vi "Panel Dryer Wilt Details.vi"(0 "Dryer In":T4 {"Night Cycle Count" format="%04d"; "Dryer Details"."Stop Dryer" items=["NO", "YES"]; "Dryer Details"."24 Hour Water Injection" items=["NO", "YES"]; "Dryer Details"."Run w/o Newfi" items=["NO", "YES"]; "Day Cycle Count" format="%04d"}, 1 "FileName":path caption="Sample Datafilename", 9 "Test State":T2) -> (4 "Dryer Details Out":T3 {"Stop Dryer" items=["NO", "YES"]; "24 Hour Water Injection" items=["NO", "YES"]; "Run w/o Newfi" items=["NO", "YES"]}, 6 "New Filenames":bool, 8 "Updated":bool, 10 "Audit Alert Out":bool)   [LabVIEW 2012]
uses:
  Dryer.ctl
  Dryer Details.ctl
  Dryer Test State.ctl
  Globals Wilt.vi
panel:
  in  "Audit Alert Button":bool
  in  "Return":bool
  out "Time":dbl[](array[numeric])
  out "Cycle Count":dbl[](array[numeric])
  in  "Tab Control":T1(tab)
  out "Dryer Details":T3 {"Stop Dryer" items=["NO", "YES"]; "24 Hour Water Injection" items=["NO", "YES"]; "Run w/o Newfi" items=["NO", "YES"]}
  out "Total Cycle Count":i32
  out "Station Number":string
  out "Status Color":u32(colorbox)
  out "Bad Com Count":i32
  out "Com Port":u8
  out "Boolean":bool
  out "Audit Alert":bool
  out "Sample Plot":cluster{dbl[], dbl[]}[](graph)
  out "Current Cycle Count":dbl
  out "I(L1),I(L2),Trmb,V.V2":dbl[][](array[numeric])
  out "Cycle Count 2":dbl[](array[numeric])
  out "Completion time":dbl[](array[numeric])
  out "L1max":dbl[](array[numeric])
  out "L2max":dbl[](array[numeric])
  out "Tmax":dbl[](array[numeric])
  out "History Plot":cluster{dbl[], dbl[]}[](graph)
  out "Serial Com Array":cluster{dbl, string}[](array[cluster]) {"?" format="%<%H:%M:%S>t"}
  out "Voltage 2":dbl[](array[numeric])
  out "Voltage":dbl[](array[numeric])
  out "Trmb":dbl[](array[numeric])
  out "L2":dbl[](array[numeric])
  out "L1":dbl[](array[numeric])
  out "Sample Record":string[][](array[string])
  out "all rows":string[][](array[string])
  in  "Read Sample Record(t, CC, Tc, \nASCII, Status, L1,L2,Trmb,V{,V2,SW} )":string[][](array[string])
  in  "Update":bool
  # "D"
  # "N"
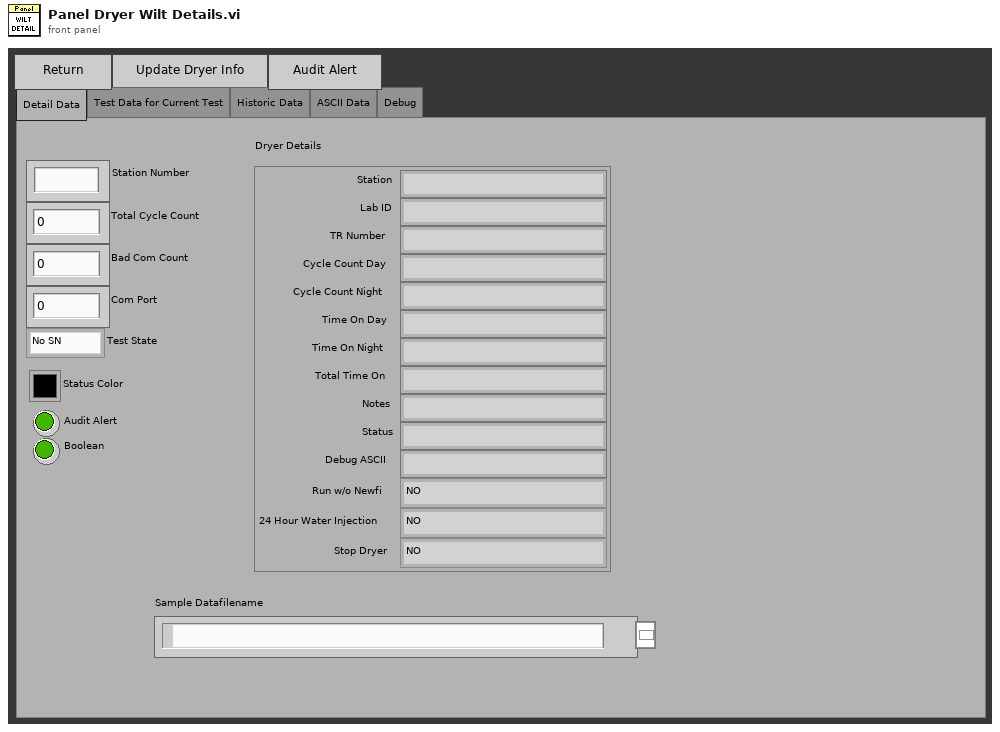
[diagram p1: front panel]
types:
  T1 = enum32{"Detail Data", "Test Data for Current Test", "Historic Data", "ASCII Data", "Debug"}
  T2 = typedef "Dryer Test State.ctl" = enum16{"No SN", "Wait Com", "Wait to Start", "Watering", "Drying", "Cooldown", "Paused", "Temp Fault", "Com Fault", "Pause Manual Station"}
  T3 = typedef "Dryer Details.ctl" = cluster{"Station":string, "Cycle Count Day":string, "Status":string, "Debug ASCII":string, "Notes":string, "Lab ID":string, "Total Time On":string, "TR Number":string, "Cycle Count Night":string, "Time On Day":string, "Time On Night":string, "Run w/o Newfi":i32, "24 Hour Water Injection":i32, "Stop Dryer":i32}
  T4 = typedef "Dryer.ctl" = cluster{"Lab ID":string, "Day Cycle Count":i32, "Station Label":string, "Dryer Details":T3, "Sample Record ":string[], "Hist Record ":string[][], "Status Color":u32, "Boolean":bool, "Com Port":u8, "Bad Com Count":i32, "Current Run Start Time":dbl, "Night Cycle Count":i32, "Station Index":i32, "Cycle Index":string, "Audit Alert":bool}
  T5 = enum16{"Read 2D Array", "Write 2D Array", "Write/Append 1D Array"}
  T6 = cluster{"FileName":path, "New File Info":bool, "Dryer In":T4, "Read Sample Record(t, CC, Tc, \nASCII, Status, L1,L2,Trmb,V{,V2,SW} )":string[][], "Audit Alert":bool, "Updated":bool}
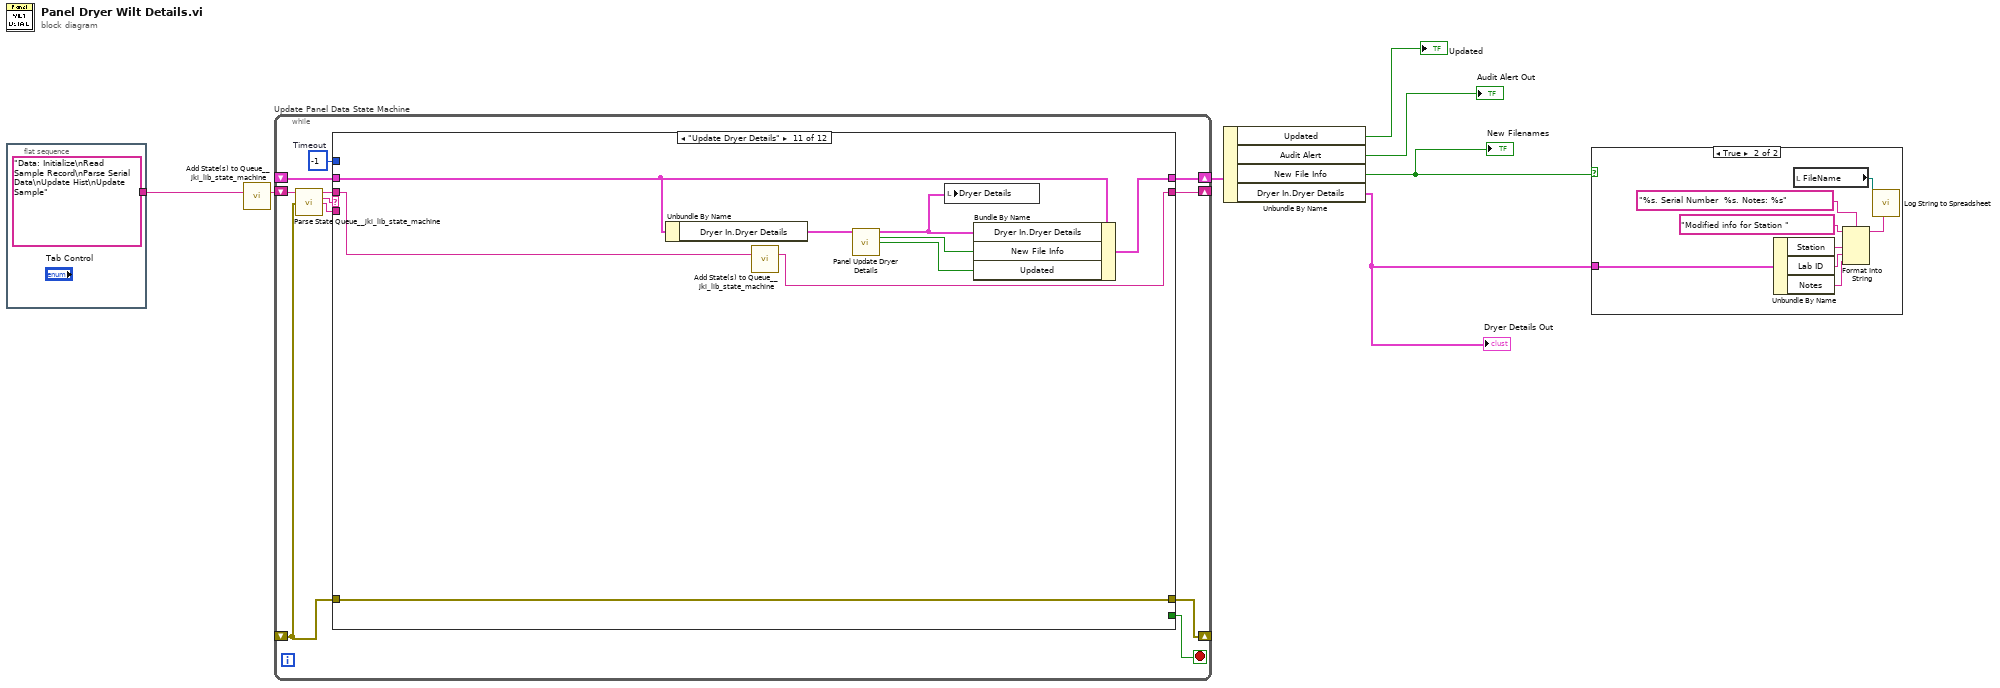
[diagram p0: block diagram]
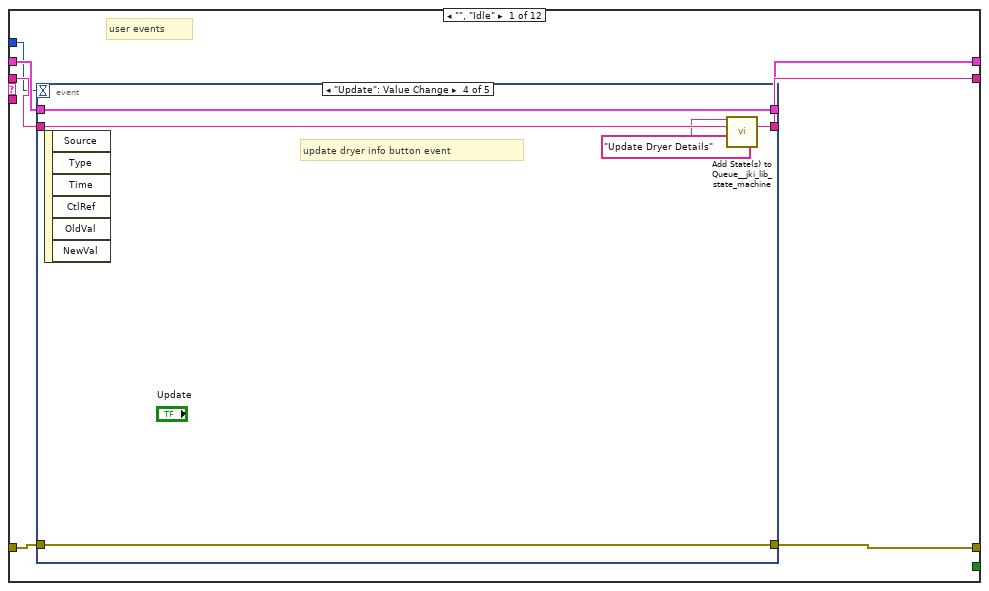
[diagram p2: hidden frame]
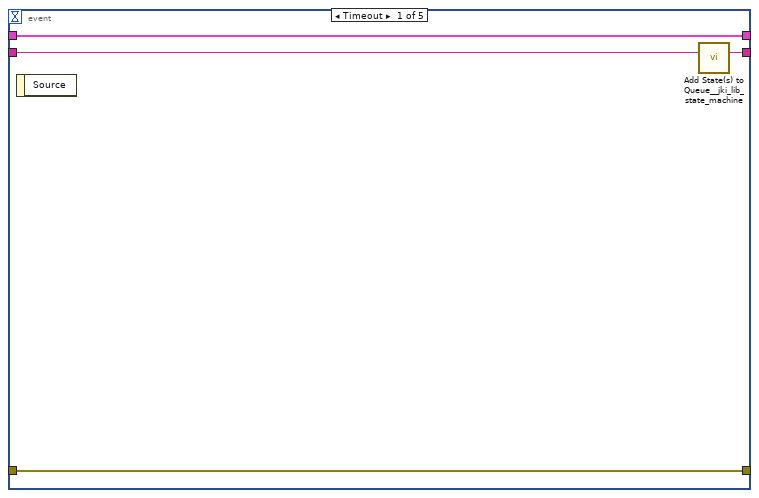
[diagram p3: hidden frame]
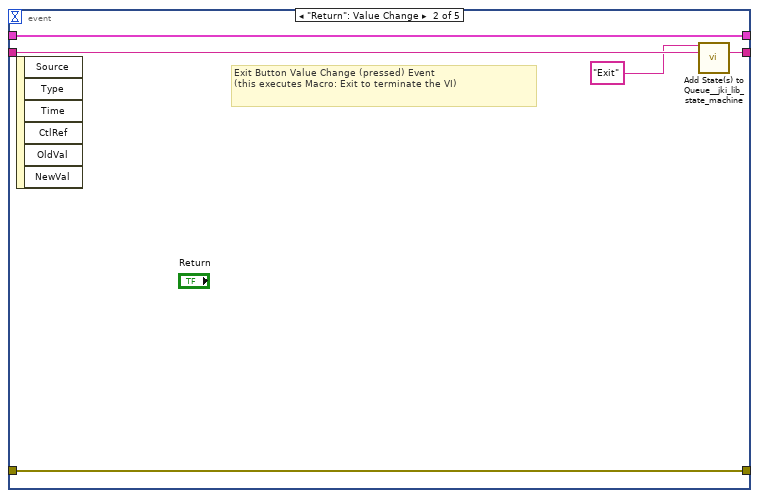
[diagram p4: hidden frame]
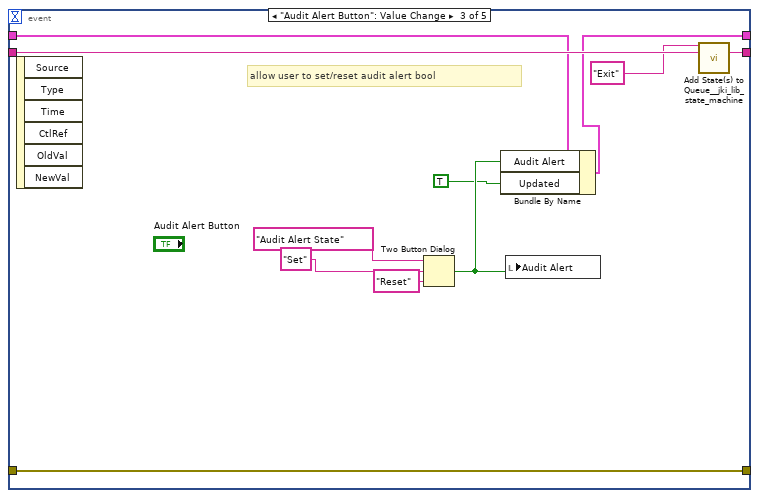
[diagram p5: hidden frame]
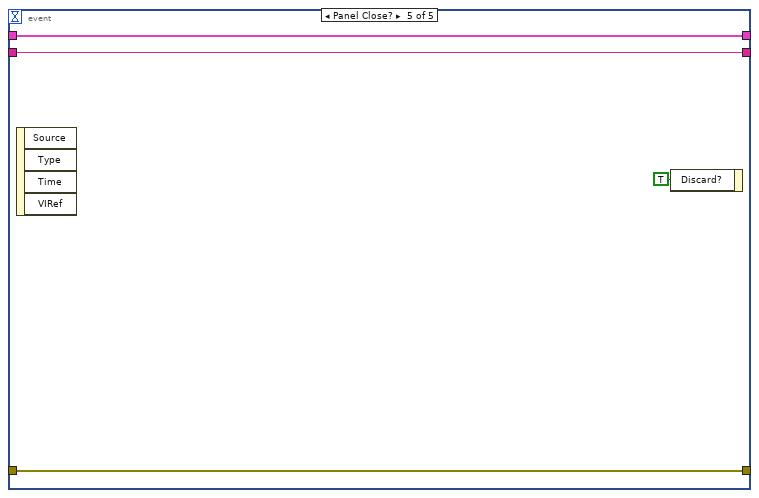
[diagram p6: hidden frame]
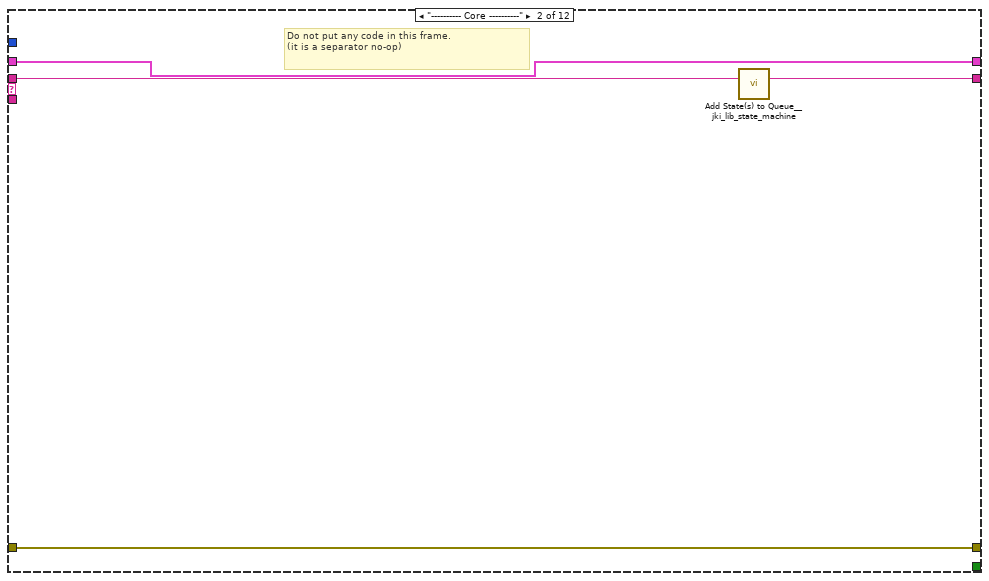
[diagram p7: hidden frame]
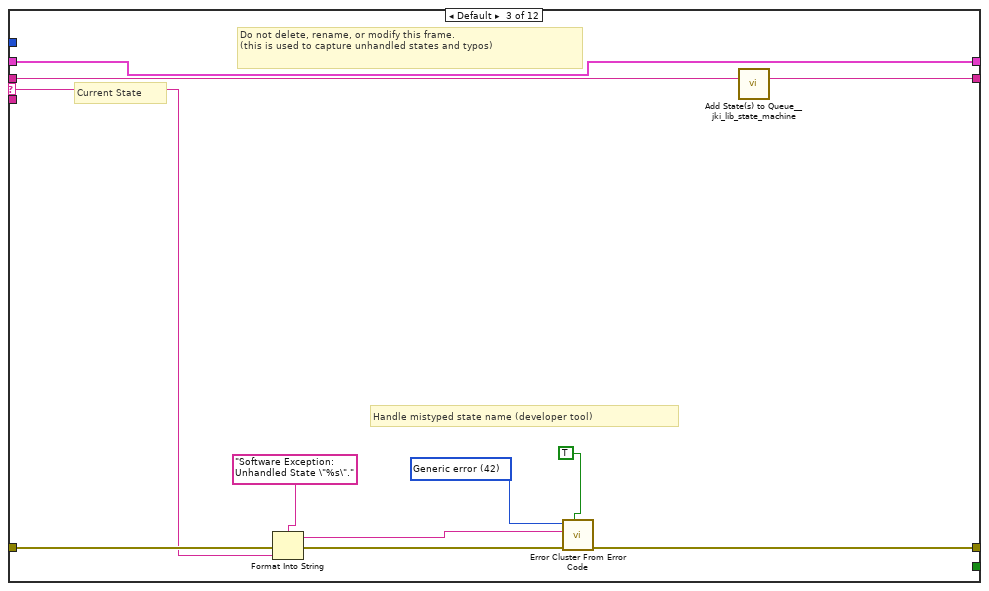
[diagram p8: hidden frame]
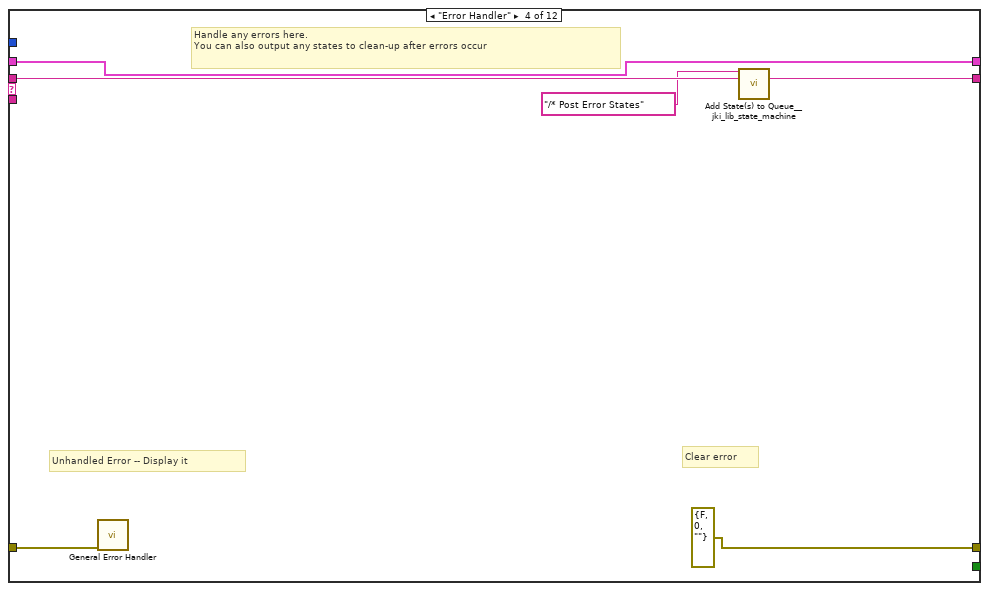
[diagram p9: hidden frame]
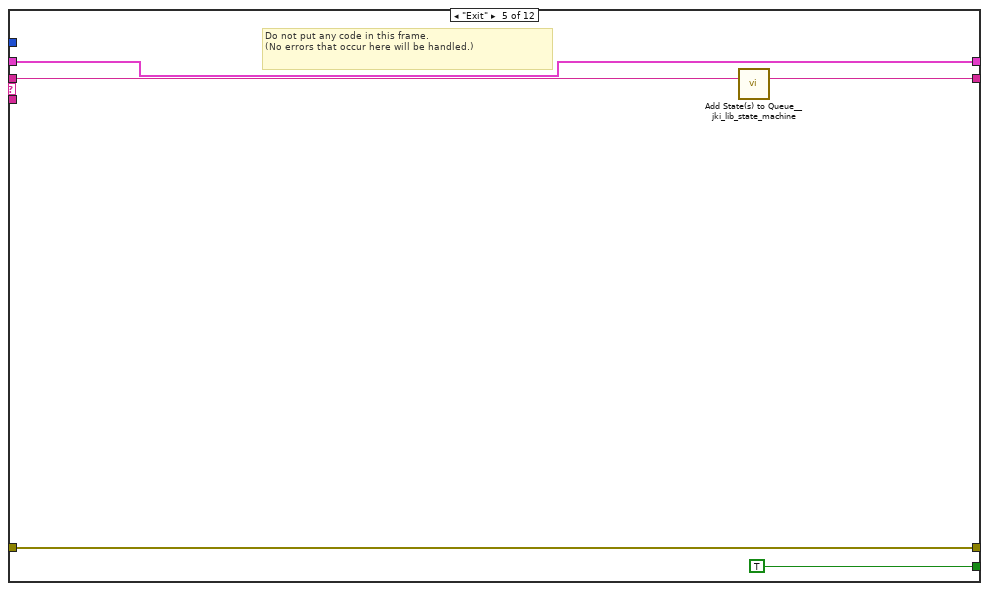
[diagram p10: hidden frame]
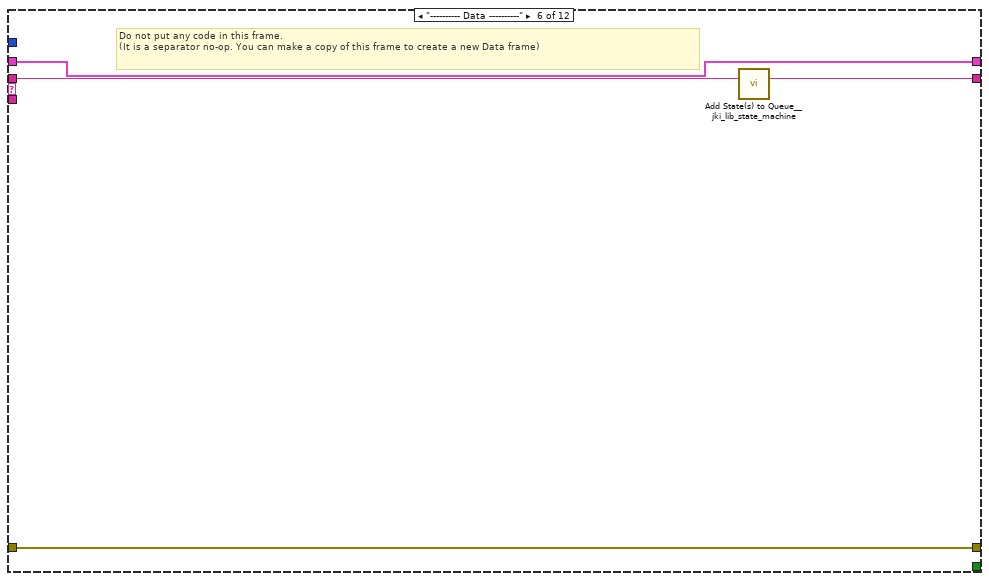
[diagram p11: hidden frame]
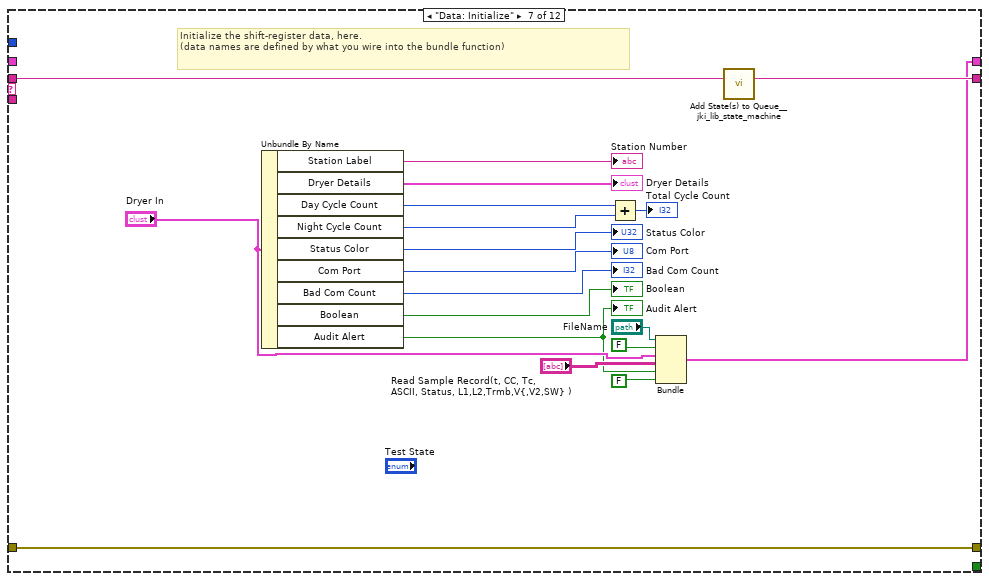
[diagram p12: hidden frame]
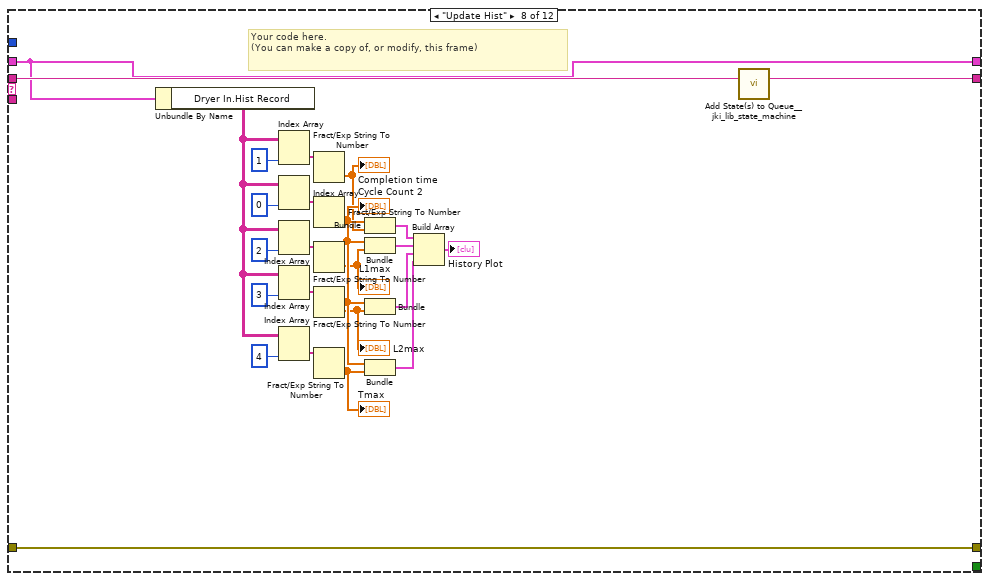
[diagram p13: hidden frame]
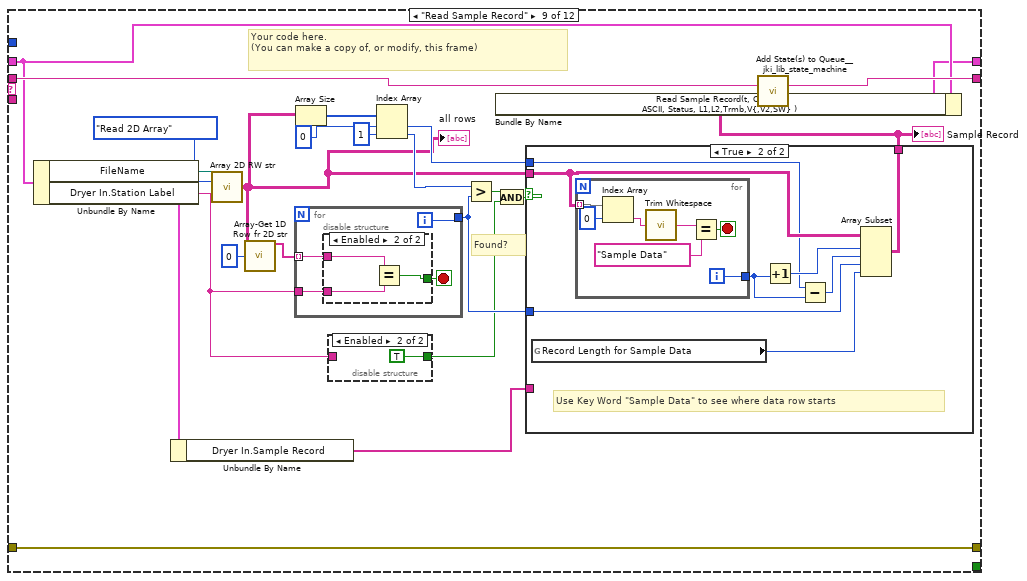
[diagram p14: hidden frame]
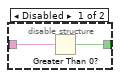
[diagram p15: hidden frame]
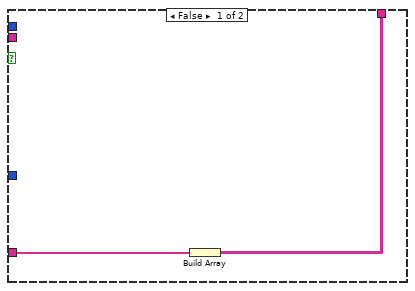
[diagram p16: hidden frame]
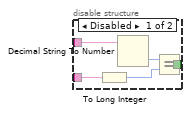
[diagram p17: hidden frame]
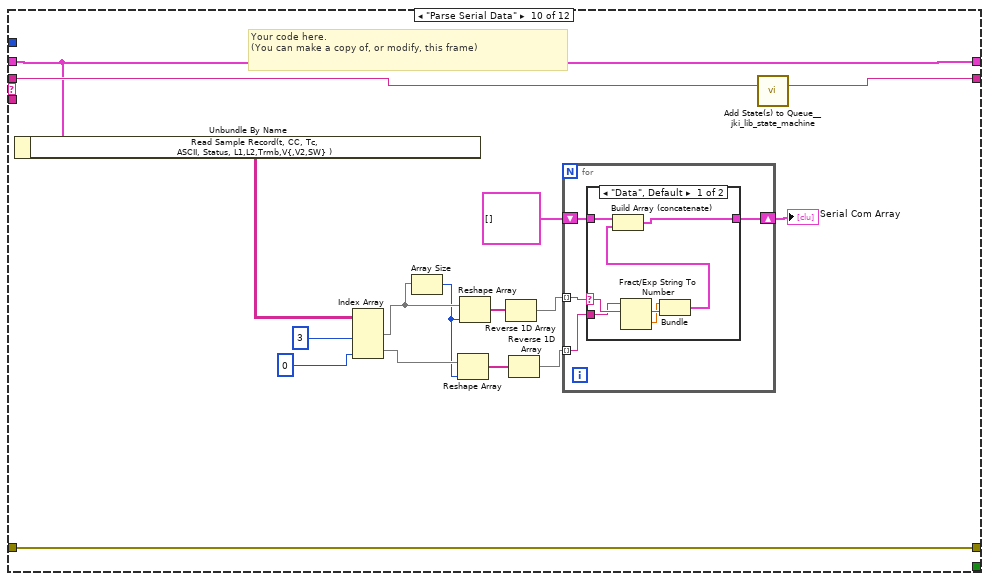
[diagram p18: hidden frame]
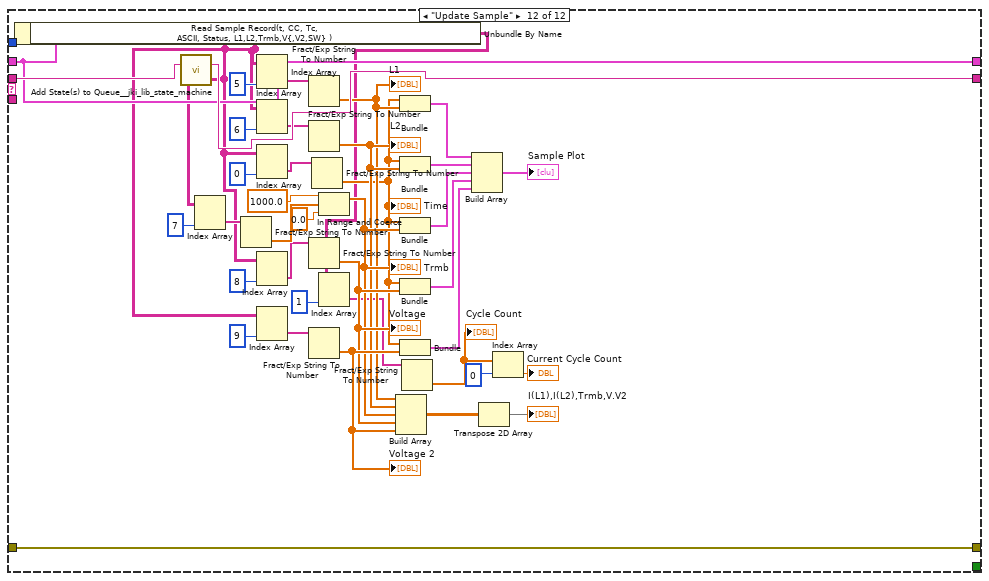
[diagram p20: hidden frame]
diagram:
  n1 = flat-sequence {
    tunnel: ["Data: Initialize\nRead Sample Record\nParse Serial Data\nUpdate Hist\nUpdate Sample"] -> w6
    frame #0 {
    }
  }
  n2 = call <vilib>:"Add State(s) to Queue__jki_lib_state_machine.vi"("State(s) in (\"\")"=w6) -> ("States Out"=w7:string)  [unwired: 14 in]
  n3 = while "Update Panel Data State Machine" {
    shift-right: [w12] -> w5
    shift-left: _ -> [w11]
    shift-right: [w15] -> _
    shift-left: _ -> [w9]
    shift-right: [w14] -> _
    shift-left: w7 -> [w16]
    stop <- w13 stop-if-true
    w10 = -1  # Timeout
    n4 = call <vilib>:"Parse State Queue__jki_lib_state_machine.vi"("State Queue"=w16, "Error In (no error)"=w9) -> ("Remaining States"=w18:string, "Current State"=w19:string, "Arguments"=w17:string)  [unwired: 11 in]
    n5 = case shown="\"Update Dryer Details\"" w19 {
      selector: w19 -> [_ _ w60 _ _ _ _ _ _ _ _ _]
      tunnel: w18 -> [w26 w59 w64 w76 w81 w85 w104 w129 w151 w199 w219 w258]
      tunnel: w17 -> [_ _ _ _ _ _ _ _ _ _ _ _]
      tunnel: w11 -> [w24 w56 w62 w73 w79 w82 _ w106 w145 w196 w215 w221]
      tunnel: [w23 w57 w66 errorcluster {"status"=FALSE, "code"=0, "source"=""} ("error out") w78 w83 w101 w127 w149 w197 w217 w256] -> w15
      tunnel: w9 -> [w22 w57 w65 w72 w78 w83 w101 w127 w149 w197 w217 w256]
      tunnel: [w25 w58 w63 w75 w80 w84 w103 w128 w150 w198 w218 w257] -> w14
      tunnel: [_ _ _ _ TRUE _ _ _ _ _ _ _] -> w13
      tunnel: [w21 w56 w62 w73 w79 w82 w102 w106 w144 w196 w214 w221] -> w12
      tunnel: w10 -> [w20 _ _ _ _ _ _ _ _ _ _ _]
      frame "", "Idle" {
        # "user events"
        n6 = event shown="[3] \"Update\": Value Change" {
          selector: _ -> [_ _ _ _ _]
          dyn-events: _ -> [_ _ _ _ _]
          timeout: w20 -> [_ _ _ _ _]
          tunnel: w26 -> [w30 w35 w46 w51 w54]
          tunnel: [w29 w34 w45 w50 w54] -> w25
          tunnel: w24 -> [w27 w32 w39 w48 w55]
          tunnel: [w28 w33 w44 w49 w52] -> w23
          tunnel: w22 -> [w28 w33 w44 w49 w52]
          tunnel: [w27 w32 w38 w48 w55] -> w21
          event Timeout {
            n7 = event-data() -> ()  [unwired: 1 in, 1 out]
            n8 = call <vilib>:"Add State(s) to Queue__jki_lib_state_machine.vi"("State(s) in (\"\")"=w30) -> ("States Out"=w29:string)  [unwired: 14 in]
          }
          event "Return": Value Change {
            # "Exit Button Value Change (pressed) Event\n(this executes Macro: Exit to terminate the VI)"
            n9 = event-data() -> ()  [unwired: 1 in, 6 out]
            n10 = call <vilib>:"Add State(s) to Queue__jki_lib_state_machine.vi"("State(s) in Front (\"\")"="Exit", "State(s) in (\"\")"=w35) -> ("States Out"=w34:string)  [unwired: 13 in]
          }
          event "Audit Alert Button": Value Change {
            # "allow user to set/reset audit alert bool"
            n11 = event-data() -> ()  [unwired: 1 in, 6 out]
            n12 = Two Button Dialog(message="Audit Alert State", 1:"Reset" ("F button name (\"Cancel\")"), 2:"Set" ("T button name (\"OK\")")) -> (T button?=w37:bool)
            n13 = Bundle By Name(cluster=w39, "Audit Alert"=w37, "Updated"=TRUE) -> (w38:T6)
            n14 = local write "Audit Alert"(w37) -> ()
            n15 = call <vilib>:"Add State(s) to Queue__jki_lib_state_machine.vi"("State(s) in Front (\"\")"="Exit", "State(s) in (\"\")"=w46) -> ("States Out"=w45:string)  [unwired: 13 in]
          }
          event "Update": Value Change {
            # "update dryer info button event"
            n16 = event-data() -> ()  [unwired: 1 in, 6 out]
            n17 = call <vilib>:"Add State(s) to Queue__jki_lib_state_machine.vi"("State(s) in Front (\"\")"="Update Dryer Details", "State(s) in (\"\")"=w51) -> ("States Out"=w50:string)  [unwired: 13 in]
          }
          event Panel Close? {
            n18 = event-data() -> ()  [unwired: 1 in, 4 out]
            n19 = event-data("Discard?"=TRUE) -> ()  [unwired: 1 in, 1 out]
          }
        }
      }
      frame "---------- Core ----------" {
        # "Do not put any code in this frame.\n(it is a separator no-op)"
        n20 = call <vilib>:"Add State(s) to Queue__jki_lib_state_machine.vi"("State(s) in (\"\")"=w59) -> ("States Out"=w58:string)  [unwired: 14 in]
      }
      frame Default {
        w69 = 42 items=["No error", "Argument error", "Memory is full", "Out of zone", "End of file", "File already open", "Generic file I/O error", "File not found", "File permission error", "Disk is full", "Duplicate path", "Too many files open", "System feature not enabled", "Resource file not found", "Cannot add resource", "Resource not found", "Image not found", "Image memory error", "Pen does not exist", "Config type invalid", "Config token not found", "Config parse error", "Config memory error", "Bad external code format", "Bad external code offset", "External code not present", "Null window", "Destroy window error", "Null menu", "Print aborted", "Bad print record", "Print driver error", "Windows error during printing", "Memory error during printing", "Print dialog error", "Generic print error", "Invalid device refnum", "Device not found", "Device parameter error", "Device unit error", "Cannot open device", "Device call aborted", "Generic error", "Cancelled by user", "Object ID too low", "Object ID too high", "Object not in heap", "Unknown heap", "Unknown object (invalid DefProc)", "Unknown object (DefProc not in table)", "Message out of range", "Invalid (null) method", "Unknown message", "Manager call not supported", "Bad address", "Network operation in progress", "Network operation timed out", "Connection is busy", "Network attribute not supported", "Network error", "Address in use", "System out of memory", "Connection aborted", "Connection refused", "Not connected", "Already connected", "Connection closed", "Initialization error (interapplication manager)", "Bad occurrence", "Wait on unbound occurrence handler", "Occurrence queue overflow", "Datalog type conflict", "Unused", "Unrecognized type (interapplication manager)", "Memory corrupt", "Failed to make temporary DLL", "Old CIN version", "Drag socket not found", "Failed to load drop-object", "Failed to register OLE object", "Failed to release OLE object", "Format specifier type mismatch", "Unknown format specifier", "Too few format specifiers", "Too many format specifiers", "Scan failed", "Newer CIN version", "Error converting to variant", "Runtime menu error", "Password tampered", "Variant attribute not found", "Incompatible variant data type", "Event data is not available", "Event Store is not present", "Occurrence is not found", "Event Queue is not created", "Event info is not available", "Refnum passed is NULL", "Error retrieving Class GUID", "Error retrieving CoClass GUID", "Error retrieving TypeLib GUID.", "Bad built application magic bytes.", "Specific driver is different from the specific driver associated with the Logical Name.", "There is no session opened to the class driver.", "Max Error", "MAX - Error with config objects", "MAX - Error loading configuration", "MAX - Group not supported"]
        # "Current State"
        # "Do not delete, rename, or modify this frame.\n(this is used to capture unhandled states and typos)"
        # "Handle mistyped state name (developer tool)"
        n21 = Format Into String(format string="Software Exception: Unhandled State \"%s\"." ("message"), error in=w65, w60) -> (resulting string=w68:string, error out=w67:errorcluster)  [unwired: 1 in]
        n22 = call <vilib>:"Error Cluster From Error Code.vi"("show call chain? (False)"=TRUE, "error in (no error)"=w67, "error message (\"\")"=w68, "error code (0)"=w69) -> ("error out"=w66:errorcluster)  [unwired: 5 in]
        n23 = call <vilib>:"Add State(s) to Queue__jki_lib_state_machine.vi"("State(s) in (\"\")"=w64) -> ("States Out"=w63:string)  [unwired: 14 in]
      }
      frame "Error Handler" {
        # "Unhandled Error -- Display it"
        # "Handle any errors here.\nYou can also output any states to clean-up after errors occur"
        # "Clear error"
        n24 = call <vilib>:"General Error Handler.vi"("error in (no error)"=w72) -> ()  [unwired: 10 in, 5 out]
        n25 = call <vilib>:"Add State(s) to Queue__jki_lib_state_machine.vi"("State(s) in Front (\"\")"="/* Post Error States", "State(s) in (\"\")"=w76) -> ("States Out"=w75:string)  [unwired: 13 in]
      }
      frame "Exit" {
        # "Do not put any code in this frame.\n(No errors that occur here will be handled.)"
        n26 = call <vilib>:"Add State(s) to Queue__jki_lib_state_machine.vi"("State(s) in (\"\")"=w81) -> ("States Out"=w80:string)  [unwired: 14 in]
      }
      frame "---------- Data ----------" {
        # "Do not put any code in this frame.\n(It is a separator no-op. You can make a copy of this frame to create a new Data frame)"
        n27 = call <vilib>:"Add State(s) to Queue__jki_lib_state_machine.vi"("State(s) in (\"\")"=w85) -> ("States Out"=w84:string)  [unwired: 14 in]
      }
      frame "Data: Initialize" {
        # "Initialize the shift-register data, here.\n(data names are defined by what you wire into the bundle function)"
        n28 = Unbundle By Name("Dryer In") -> ("Station Label"=→"Station Number":string, "Dryer Details"=→"Dryer Details":T3, "Day Cycle Count"=w90:i32, "Night Cycle Count"=w89:i32, "Status Color"=→"Status Color":u32, "Com Port"=→"Com Port":u8, "Bad Com Count"=→"Bad Com Count":i32, "Boolean"=→"Boolean":bool, "Audit Alert"=w87:bool)
        "Audit Alert" <- w87
        n29 = Add(x=w90, y=w89) -> (x+y=→"Total Cycle Count":i32)
        n30 = Bundle("FileName"="FileName", "New File Info"=FALSE, "Dryer In"="Dryer In", "Read Sample Record(t, CC, Tc, \nASCII, Status, L1,L2,Trmb,V{,V2,SW} )"="Read Sample Record(t, CC, Tc, \nASCII, Status, L1,L2,Trmb,V{,V2,SW} )", "Audit Alert"=w87, "Updated"=FALSE) -> (w102:T6)  [unwired: 1 in]
        n31 = call <vilib>:"Add State(s) to Queue__jki_lib_state_machine.vi"("State(s) in (\"\")"=w104) -> ("States Out"=w103:string)  [unwired: 14 in]
      }
      frame "Update Hist" {
        # "Your code here.\n(You can make a copy of, or modify, this frame)"
        n32 = Unbundle By Name(w106) -> ("Dryer In.Hist Record"=w105:string[][])
        n33 = Index Array(array=w105, index (col)=1 ("disabled index (col)")) -> (element=w109:string[])  [unwired: 1 in]
        n34 = Index Array(array=w105, index (col)=0 ("disabled index (col)")) -> (element=w107:string[])  [unwired: 1 in]
        n35 = Index Array(array=w105, index (col)=2 ("disabled index (col)")) -> (element=w110:string[])  [unwired: 1 in]
        n36 = Index Array(array=w105, index (col)=3 ("disabled index (col)")) -> (element=w114:string[])  [unwired: 1 in]
        n37 = Index Array(array=w105, index (col)=4 ("disabled index (col)")) -> (element=w123:string[])  [unwired: 1 in]
        n38 = Fract/Exp String To Number(string=w109) -> (number=w115:dbl[])  [unwired: 3 in, 1 out]
        "Completion time" <- w115
        n39 = Fract/Exp String To Number(string=w107) -> (number=w125:dbl[])  [unwired: 3 in, 1 out]
        "Cycle Count 2" <- w125
        n40 = Fract/Exp String To Number(string=w110) -> (number=w116:dbl[])  [unwired: 3 in, 1 out]
        "L1max" <- w116
        n41 = Fract/Exp String To Number(string=w114) -> (number=w117:dbl[])  [unwired: 3 in, 1 out]
        "L2max" <- w117
        n42 = Fract/Exp String To Number(string=w123) -> (number=w124:dbl[])  [unwired: 3 in, 1 out]
        "Tmax" <- w124
        n43 = Bundle(w125, w115) -> (w119:cluster{dbl[], dbl[]})  [unwired: 1 out]
        n44 = Bundle(w125, w116) -> (w120:cluster{dbl[], dbl[]})  [unwired: 1 out]
        n45 = Bundle(w125, w117) -> (w121:cluster{dbl[], dbl[]})  [unwired: 1 out]
        n46 = Bundle(w125, w124) -> (w126:cluster{dbl[], dbl[]})  [unwired: 1 out]
        n47 = Build Array(w119, w120, w121, w126) -> (→"History Plot":cluster{dbl[], dbl[]}[])
        n48 = call <vilib>:"Add State(s) to Queue__jki_lib_state_machine.vi"("State(s) in (\"\")"=w129) -> ("States Out"=w128:string)  [unwired: 14 in]
      }
      frame "Read Sample Record" {
        # "Found?"
        # "Your code here.\n(You can make a copy of, or modify, this frame)"
        n49 = Unbundle By Name(w145) -> ("FileName"=w132:path, "Dryer In.Station Label"=w140:string)
        n50 = Unbundle By Name(w145) -> ("Dryer In.Sample Record"=w138:string[])
        n51 = call "Array 2D RW str.vi"("file path (dialog if empty)"=w132, "Write/Read"=T5."Read 2D Array") -> ("Read all rows"=w131:string[][])  [unwired: 13 in]
        "all rows" <- w131
        n52 = call "Array-Get 1D Row fr 2D str.vi"("all rows"=w131, "row index"=0) -> ("row"=w135:string[])  [unwired: 13 in]
        n53 = for {
          tunnel: w135 -> [w175] mode=indexing
          tunnel: w140 -> [w174]
          tunnel: [w172] -> w146
          i -> [w172]
          stop <- w173 stop-if-true
          n54 = disable-structure shown="Enabled" {
            disable-tunnel: w175 -> [w180 w182]
            disable-tunnel: w174 -> [w178 w183]
            disable-tunnel: [w176 w181] -> w173
            frame Disabled {
              n55 = To Long Integer(number=w178) -> (32bit integer=w177:i32)
              n56 = Decimal String To Number(string=w180) -> (number=w179:i32)  [unwired: 2 in, 1 out]
              n57 = Equal?(x=w179, y=w177) -> (x = y?=w176:bool)
            }
            frame Enabled {
              n58 = Equal?(x=w182, y=w183) -> (x = y?=w181:bool)
            }
          }
        }
        n59 = Array Size(array=w131) -> (size(s)=w148:i32[])
        n60 = disable-structure shown="Enabled" {
          disable-tunnel: w140 -> [w153 _]
          disable-tunnel: [w152 TRUE] -> w139
          frame Disabled {
            n61 = Greater Than 0?(x=w153) -> (x > 0?=w152:bool)
          }
          frame Enabled {
          }
        }
        n62 = Index Array(array=w148, index #1=0 ("index"), index #2=1 ("index")) -> (element #1=w133:i32, element #2=w136:i32)
        n63 = Greater?(x=w136, y=w146) -> (0:w142:bool)
        n64 = And(x=w142, y=w139) -> (x .and. y?=w141:bool)
        n65 = case shown="True" w141 {
          tunnel: w131 -> [_ w163]
          tunnel: w146 -> [_ w162]
          tunnel: [w155 w161] -> w143
          tunnel: w138 -> [w156 _]
          tunnel: w133 -> [_ w158]
          frame False {
            n66 = Build Array(w156) -> (w155:string[][])
          }
          frame True {
            # "Use Key Word \"Sample Data\" to see where data row starts"
            n67 = global read "Globals Wilt.vi" "Record Length for Sample Data"() -> (w160:i32)
            n68 = for {
              tunnel: w163 -> [w171] mode=indexing
              tunnel: [w168] -> w157
              i -> [w168]
              stop <- w167 stop-if-true
              n69 = Index Array(array=w171, index=0) -> (element=w166:string)
              n70 = call <vilib>:"Trim Whitespace.vi"("string"=w166) -> ("trimmed string"=w165:string)  [unwired: 1 in]
              n71 = Equal?(x=w165, y="Sample Data") -> (x = y?=w167:bool)
            }
            n72 = Increment(x=w157) -> (x+1=w164:i32)
            n73 = Subtract(x=w158, y=w157) -> (x-y=w159:i32)
            n74 = Array Subset(array=w163, index (row)=w164, length (row)=w159, index (col)=w162, length (col)=w160) -> (w161:string[][])
          }
        }
        "Sample Record" <- w143
        n75 = Bundle By Name(cluster=w145, "Read Sample Record(t, CC, Tc, \nASCII, Status, L1,L2,Trmb,V{,V2,SW} )"=w143) -> (w144:T6)
        n76 = call <vilib>:"Add State(s) to Queue__jki_lib_state_machine.vi"("State(s) in (\"\")"=w151) -> ("States Out"=w150:string)  [unwired: 14 in]
      }
      frame "Parse Serial Data" {
        # "Your code here.\n(You can make a copy of, or modify, this frame)"
        n77 = Unbundle By Name(w196) -> ("Read Sample Record(t, CC, Tc, \nASCII, Status, L1,L2,Trmb,V{,V2,SW} )"=w186:string[][])
        n78 = Index Array(array=w186, index (col) #1=3 ("disabled index (col)"), index (col) #2=0 ("index (col)")) -> (element #1=w185:string[], element #2=w192:string[])  [unwired: 2 in]
        n79 = Array Size(array=w185) -> (size(s)=w184:i32)
        n80 = Reshape Array(w192, w184) -> (w191:string[])
        n81 = Reshape Array(w185, w184) -> (w194:string[])
        n82 = Reverse 1D Array(array=w194) -> (reversed array=w190:string[])
        n83 = Reverse 1D Array(array=w191) -> (reversed array=w189:string[])
        n84 = for {
          tunnel: w190 -> [w203] mode=indexing
          tunnel: w189 -> [w202] mode=indexing
          shift-right: [w201] -> w188
          shift-left: cluster{dbl, string}[] [] -> [w200]
          n85 = case shown="\"Data\", Default" w203 {
            selector: w203 -> [w209 _]
            tunnel: w202 -> [w208 _]
            tunnel: [w206 w210] -> w201
            tunnel: w200 -> [w205 w210]
            frame "Data", Default {
              n86 = Fract/Exp String To Number(string=w208) -> (number=w204:dbl)  [unwired: 3 in, 1 out]
              n87 = Bundle(w204, w209) -> (w207:cluster{dbl, string})  [unwired: 1 in]
              n88 = Build Array (concatenate)(w205, w207) -> (w206:cluster{dbl, string}[])
            }
            frame "" {
            }
          }
        }
        "Serial Com Array" <- w188
        n89 = call <vilib>:"Add State(s) to Queue__jki_lib_state_machine.vi"("State(s) in (\"\")"=w199) -> ("States Out"=w198:string)  [unwired: 14 in]
      }
      frame "Update Dryer Details" {
        n90 = Unbundle By Name(w215) -> ("Dryer In.Dryer Details"=w216:T3)
        n91 = call <vilib>:"Add State(s) to Queue__jki_lib_state_machine.vi"("State(s) in (\"\")"=w219) -> ("States Out"=w218:string)  [unwired: 14 in]
        n92 = call "Panel Update Dryer Details.vi"("Dryer Details In"=w216) -> ("Dryer Details Out"=w212:T3, "New Filenames"=w213:bool, "Updated"=w211:bool)  [unwired: 12 in]
        n93 = local write "Dryer Details"(w212) -> ()
        n94 = Bundle By Name(cluster=w215, "Dryer In.Dryer Details"=w212, "New File Info"=w213, "Updated"=w211) -> (w214:T6)
      }
      frame "Update Sample" {
        n95 = Unbundle By Name(w221) -> ("Read Sample Record(t, CC, Tc, \nASCII, Status, L1,L2,Trmb,V{,V2,SW} )"=w220:string[][])
        n96 = call <vilib>:"Add State(s) to Queue__jki_lib_state_machine.vi"("State(s) in (\"\")"=w258) -> ("States Out"=w257:string)  [unwired: 14 in]
        n97 = Index Array(array=w220, index (col)=7 ("disabled index (col)")) -> (element=w230:string[])  [unwired: 1 in]
        n98 = Fract/Exp String To Number(string=w230) -> (number=w246:dbl[])  [unwired: 3 in, 1 out]
        n99 = Index Array(array=w220, index (col)=5 ("disabled index (col)")) -> (element=w225:string[])  [unwired: 1 in]
        n100 = Index Array(array=w220, index (col)=6 ("disabled index (col)")) -> (element=w227:string[])  [unwired: 1 in]
        n101 = Index Array(array=w220, index (col)=0 ("disabled index (col)")) -> (element=w223:string[])  [unwired: 1 in]
        n102 = Index Array(array=w220, index (col)=8 ("disabled index (col)")) -> (element=w232:string[])  [unwired: 1 in]
        n103 = Index Array(array=w220, index (col)=9 ("disabled index (col)")) -> (element=w234:string[])  [unwired: 1 in]
        n104 = Fract/Exp String To Number(string=w225) -> (number=w249:dbl[])  [unwired: 3 in, 1 out]
        "L1" <- w249
        n105 = Fract/Exp String To Number(string=w227) -> (number=w250:dbl[])  [unwired: 3 in, 1 out]
        "L2" <- w250
        n106 = Fract/Exp String To Number(string=w232) -> (number=w252:dbl[])  [unwired: 3 in, 1 out]
        "Voltage" <- w252
        n107 = Fract/Exp String To Number(string=w234) -> (number=w253:dbl[])  [unwired: 3 in, 1 out]
        "Voltage 2" <- w253
        n108 = Fract/Exp String To Number(string=w223) -> (number=w236:dbl[])  [unwired: 3 in, 1 out]
        "Time" <- w236
        n109 = In Range and Coerce(upper limit=1000.0 ("String"), x=w246, lower limit=0.0 ("String")) -> (coerced(x)=w251:dbl[])  [unwired: 1 out]
        "Trmb" <- w251
        n110 = Index Array(array=w220, index (col)=1 ("disabled index (col)")) -> (element=w224:string[])  [unwired: 1 in]
        n111 = Build Array(w249, w250, w251, w252, w253) -> (w254:dbl[][])
        n112 = Bundle(w236, w249) -> (w238:cluster{dbl[], dbl[]})  [unwired: 1 out]
        n113 = Bundle(w236, w250) -> (w237:cluster{dbl[], dbl[]})  [unwired: 1 out]
        n114 = Bundle(w236, w251) -> (w239:cluster{dbl[], dbl[]})  [unwired: 1 out]
        n115 = Bundle(w236, w252) -> (w240:cluster{dbl[], dbl[]})  [unwired: 1 out]
        n116 = Bundle(w236, w253) -> (w241:cluster{dbl[], dbl[]})  [unwired: 1 out]
        n117 = Fract/Exp String To Number(string=w224) -> (number=w243:dbl[])  [unwired: 3 in, 1 out]
        "Cycle Count" <- w243
        n118 = Build Array(w238, w237, w239, w240, w241) -> (→"Sample Plot":cluster{dbl[], dbl[]}[])
        n119 = Transpose 2D Array(2D array=w254) -> (transposed array=→"I(L1),I(L2),Trmb,V.V2":dbl[][])
        n120 = Index Array(array=w243, index=0) -> (element=→"Current Cycle Count":dbl)
      }
    }
  }
  n121 = Unbundle By Name(w5) -> ("Updated"=→"Updated":bool, "Audit Alert"=→"Audit Alert Out":bool, "New File Info"=w3:bool, "Dryer In.Dryer Details"=w4:T3)
  "Dryer Details Out" <- w4
  "New Filenames" <- w3
  n122 = case shown="True" w3 {
    tunnel: w4 -> [_ w265]
    frame False {
    }
    frame True {
      n123 = Unbundle By Name(w265) -> ("Station"=w264:string, "Lab ID"=w262:string, "Notes"=w261:string)
      n124 = local read "FileName"() -> (w259:path)
      n125 = Format Into String(format string="%s. Serial Number  %s. Notes: %s", initial string="Modified info for Station ", w264, w262, w261) -> (resulting string=w260:string)  [unwired: 1 in, 1 out]
      n126 = call "Log String to Spreadsheet.vi"("String"=w260, "FileName"=w259) -> ()  [unwired: 9 in, 1 out]
    }
  }
